vi "rqcAlice Modulator (FPGA).vi"(0 "pulse arrived":bool, 2 "reset":bool, 7 "DAC random level":u8, 9 "rqcAlice PM.config":T1) -> (4 "DAC level":u8, 10 "DAC value changed":bool=TRUE)   [LabVIEW 2018]
uses:
  Custom Controls/Phase Modulator/rqcAlice Mod.Config.ctl
  <vilib>/RQC/FPGA Basic Logic/Counters/Counter (U8).vi
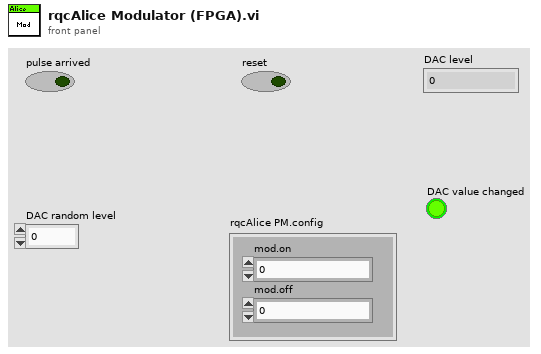
[diagram p1: front panel]
types:
  T1 = typedef "rqcAlice Mod.Config.ctl" = cluster{"mod.on":u8, "mod.off":u8}
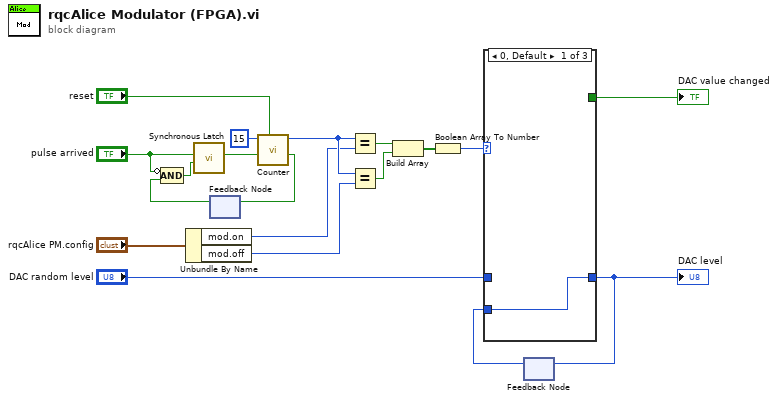
[diagram p0: block diagram]
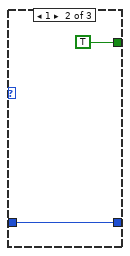
[diagram p2: hidden frame]
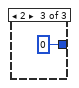
[diagram p3: hidden frame]
diagram:
  n1 = Unbundle By Name("rqcAlice PM.config") -> ("mod.on"=w9:u8, "mod.off"=w8:u8)
  n2 = feedback #1() -> (w15:bool)  [unwired: 1 in]
  n3 = Compound Arithmetic op=AND(invert "pulse arrived", w15) -> (w17:bool)
  n4 = call <vilib>:"Synchronous Latch.vi"("clear"=w17, "set"="pulse arrived") -> ("out"=w18:bool)  [unwired: 9 in]
  n5 = call-poly <vilib>:"Counter.vi"("reset"="reset", "increment"=w18, "bound"=u8 15) -> ("done"=w16:bool, "count out"=w14:u8)  [unwired: 7 in]
  n6 = feedback-in #1(w16) -> ()
  n7 = Equal?(x=w14, y=w9) -> (x = y?=w5:bool)
  n8 = Equal?(x=w14, y=w8) -> (x = y?=w13:bool)
  n9 = Build Array(w5, w13) -> (w11:bool[])
  n10 = Boolean Array To Number(Boolean array=w11) -> (number=w12:u8)
  n11 = feedback #2() -> (w6:u8)  [unwired: 1 in]
  n12 = case shown="0, Default" w12 {
    tunnel: [w20 w21 u8 0 ("DAC random level")] -> w7
    tunnel: w6 -> [w20 _ _]
    tunnel: [_ TRUE _] -> w4
    tunnel: "DAC random level" -> [_ w21 _]
    frame 0, Default {
    }
    frame 1 {
    }
    frame 2 {
    }
  }
  "DAC level" <- w7
  "DAC value changed" <- w4
  n13 = feedback-in #2(w7) -> ()
